vi "MagnetArduinoVoltageReader.vi"(7 "Aux Field Range (Oe)":dbl, 8 "error in (no error)":errorcluster, 9 "Aux max voltage (mV)":dbl, 10 "Hall probe/Aux":bool, 11 "VISA Refnum in":refnum<visa-resource-name>) -> (0 "error out":errorcluster, 2 "Numeric":dbl, 3 "VISA Refnum out":refnum<visa-resource-name>)   [LabVIEW 2017, in "Fridge Software v2.1.lvlib"]
uses:
  Fridge Software v2.1.lvlib
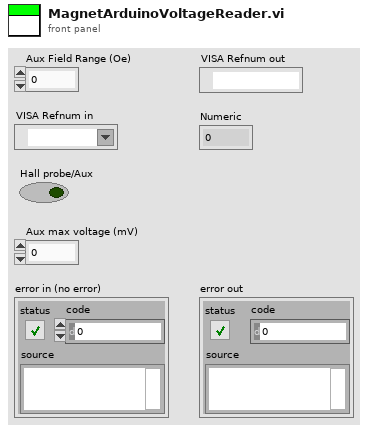
[diagram p1: front panel]
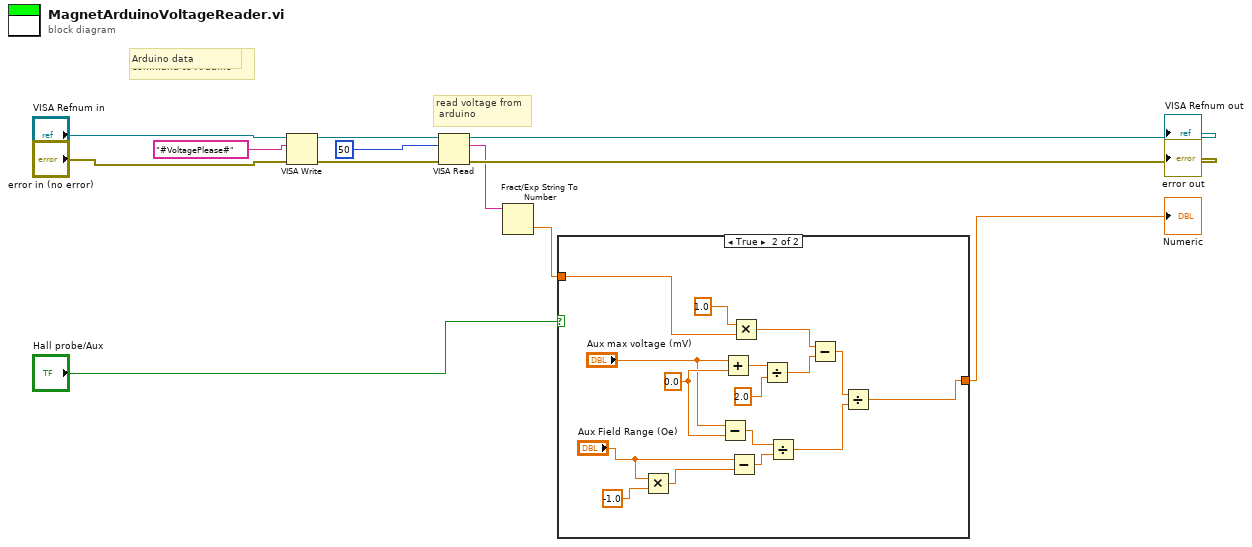
[diagram p0: block diagram]
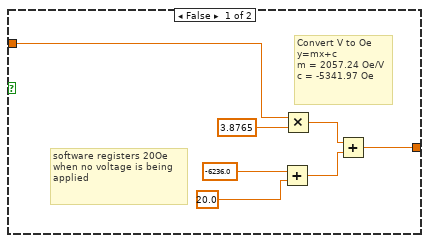
[diagram p2: hidden frame]
diagram:
  # "Arduino data"
  # "read voltage from\n arduino"
  # "Write voltage read command to Arduino"
  n1 = VISA Write(VISA resource name="VISA Refnum in", write buffer="#VoltagePlease#" ("Send to Arduino"), error in (no error)="error in (no error)") -> (VISA resource name out=w3:refnum<visa-resource-name>, error out=w6:errorcluster)  [unwired: 1 out]
  n2 = VISA Read(VISA resource name=w3, byte count=u32 50 ("milliseconds to wait"), error in (no error)=w6) -> (VISA resource name out=→"VISA Refnum out":refnum<visa-resource-name>, read buffer=w1:string, error out=→"error out":errorcluster)  [unwired: 1 out]
  n3 = Fract/Exp String To Number(string=w1) -> (number=w10:dbl)  [unwired: 3 in, 1 out]
  n4 = case shown="True" "Hall probe/Aux" {
    tunnel: w10 -> [w14 w27]
    tunnel: [w13 w24] -> w11
    frame False {
      # "software registers 20Oe when no voltage is being applied"
      # "Convert V to Oe\ny=mx+c\nm = 2057.24 Oe/V\nc = -5341.97 Oe"
      n5 = Add(x=-6236.0, y=20.0) -> (x+y=w18:dbl)
      n6 = Multiply(x=w14, y=3.8765) -> (x*y=w19:dbl)
      n7 = Add(x=w19, y=w18) -> (x+y=w13:dbl)
    }
    frame True {
      w32 = 0.0
      n8 = Multiply(x="Aux Field Range (Oe)", y=-1.0) -> (x*y=w22:dbl)
      n9 = Subtract(x="Aux max voltage (mV)", y=w32) -> (x-y=w31:dbl)
      n10 = Add(x="Aux max voltage (mV)", y=w32) -> (x+y=w35:dbl)
      n11 = Subtract(x="Aux Field Range (Oe)", y=w22) -> (x-y=w30:dbl)
      n12 = Multiply(x=1.0, y=w27) -> (x*y=w25:dbl)
      n13 = Divide(x=w35, y=2.0) -> (x/y=w33:dbl)
      n14 = Divide(x=w31, y=w30) -> (x/y=w28:dbl)
      n15 = Subtract(x=w25, y=w33) -> (x-y=w29:dbl)
      n16 = Divide(x=w29, y=w28) -> (x/y=w24:dbl)
    }
  }
  "Numeric" <- w11
